vi "Write Resource Name.vi"(8 "error in (no error)":errorcluster, 10 "Resource Name":string, 11 "Abstract Switch Init Parameters in":refnum<class "Abstract Switch Init Parameters.lvclass">) -> (0 "error out":errorcluster, 3 "Abstract Switch Init Parameters out":refnum<class "Abstract Switch Init Parameters.lvclass">)   [LabVIEW 2027, in "Messaging.lvlib" / "Abstract Switch Init Parameters.lvclass"]
uses:
  Abstract Switch Init Parameters.lvclass
  Abstract Switch Init Parameters.lvclass/Abstract Switch Init Parameters.ctl
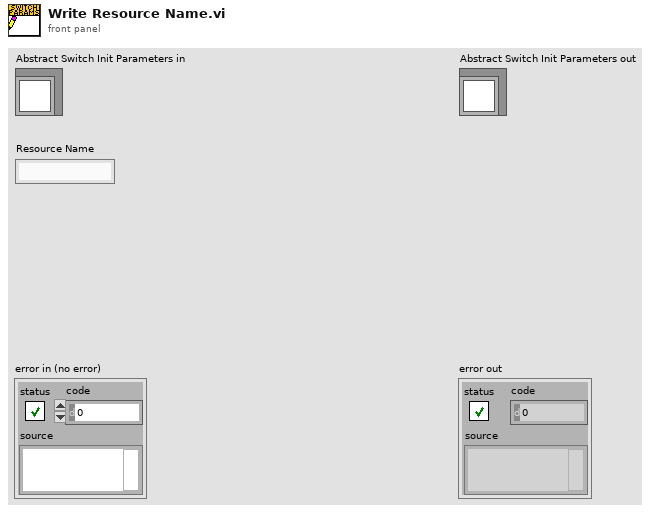
[diagram p1: front panel]
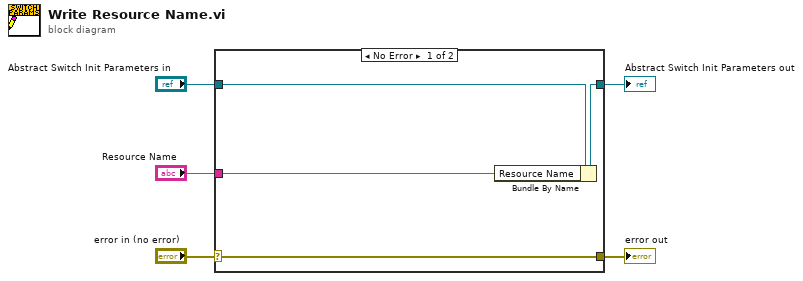
[diagram p0: block diagram]
diagram:
  n1 = case shown="No Error" "error in (no error)" {
    selector: "error in (no error)" -> [w9 w10]
    tunnel: [w9 w10] -> w4
    tunnel: [w7 w11] -> w2
    tunnel: "Abstract Switch Init Parameters in" -> [w8 w11]
    tunnel: "Resource Name" -> [w6 _]
    frame No Error {
      n2 = Bundle By Name(cluster=w8, "Resource Name"=w6) -> (w7:refnum<class "Abstract Switch Init Parameters.lvclass">)
    }
    frame Error {
    }
  }
  "error out" <- w4
  "Abstract Switch Init Parameters out" <- w2
